vi "GetPressureAtMouse.vi"(2 "Coords":T1, 3 "GraphRefnum":refnum<vi>) -> (0 "Numeric":dbl, 1 "String":string)   [LabVIEW 2013, in "main.lvlib"]
uses:
  main.lvlib
  <vilib>/Utility/miscctls.llb/LVPoint32TypeDef.ctl
  Controls/Enum Globals.ctl
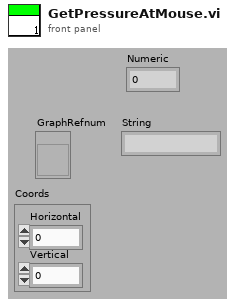
[diagram p1: front panel]
types:
  T1 = typedef "LVPoint32TypeDef.ctl" = cluster{"Horizontal":i32, "Vertical":i32}
  T2 = typedef "main.lvlib/Enum Globals.ctl" = enum16{"Init", "Set DataPath", "Set Freq", "Get"}
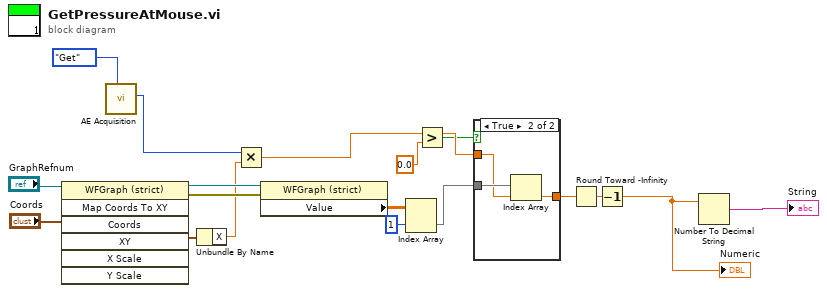
[diagram p0: block diagram]
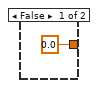
[diagram p2: hidden frame]
diagram:
  n1 = invoke class="WFGraph (strict)" method="Map Coords To XY"(reference="GraphRefnum", "Coords"="Coords") -> (reference out=w15:refnum<vi>, error out=w16:errorcluster, "XY"=w13:cluster{"X":dbl, "Y":dbl})  [unwired: 5 in, 4 out]
  n2 = call "AE Acquisition.vi"("Action"=Enum_Globals."Get") -> ("Freq Out"=w3:i32)  [unwired: 7 in, 3 out]
  n3 = Unbundle By Name(w13) -> ("X"=w14:dbl)
  n4 = Multiply(x=w3, y=w14) -> (x*y=w8:dbl)
  n5 = property class="WFGraph (strict)"(reference=w15, error in=w16) -> ("Value"=w9:dbl[][])  [unwired: 2 out]
  n6 = Index Array(array=w9, index (row)=1) -> (element=w11:dbl[])  [unwired: 1 in]
  n7 = Greater?(x=w8, y=0.0) -> (0:w6:bool)
  n8 = case shown="True" w6 {
    tunnel: w11 -> [_ w22]
    tunnel: w8 -> [_ w21]
    tunnel: [0.0 w20] -> w12
    frame False {
    }
    frame True {
      n9 = Index Array(array=w22, index=w21) -> (element=w20:dbl)
    }
  }
  n10 = Round Toward -Infinity(1:w12) -> (0:w2:dbl)
  n11 = Decrement(x=w2) -> (x-1=w1:dbl)
  "Numeric" <- w1
  n12 = Number To Decimal String(number=w1) -> (decimal integer string=→"String":string)  [unwired: 1 in]
